vi "GetState.vi"(8 "State In":T1, 11 "QueueIn":refnum<queue>) -> (0 "State Out":T1, 1 "Parameter":string, 2 "State":string, 3 "QueueOut":refnum<queue>)   [LabVIEW 2016]
uses:
  Controls/StateData.ctl
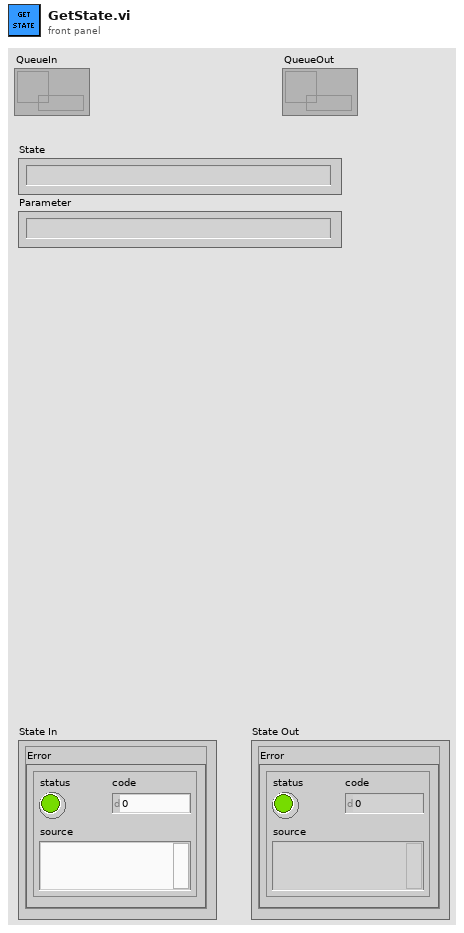
[diagram p1: front panel]
types:
  T1 = typedef "StateData.ctl" = cluster{"Error":errorcluster}
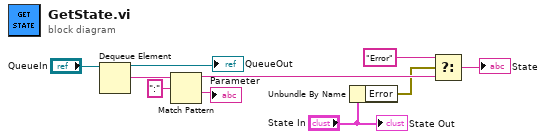
[diagram p0: block diagram]
diagram:
  n1 = Dequeue Element(queue="QueueIn") -> (queue out=→"QueueOut":refnum<queue>, element=w10:string)  [unwired: 2 in, 2 out]
  n2 = Match Pattern(string=w10, regular expression=":") -> (before substring=w5:string, after substring=→"Parameter":string)  [unwired: 1 in, 2 out]
  n3 = Unbundle By Name("State In") -> ("Error"=w2:errorcluster)
  n4 = Select(t="Error", s=w2, f=w5) -> (s? t:f=→"State":string)
  "State Out" <- "State In"
